vi "WM Period-Depth to Wave Length.vi"(1 "Water Depth":dbl=0.01 min=0.01 step=0.01 format="%.2f", 2 "Period":dbl=0.01 min=0.01 format="%.2f") -> (0 "WaveLength":dbl format="%.4f")   [LabVIEW 2012]
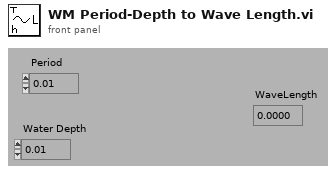
[diagram p1: front panel]
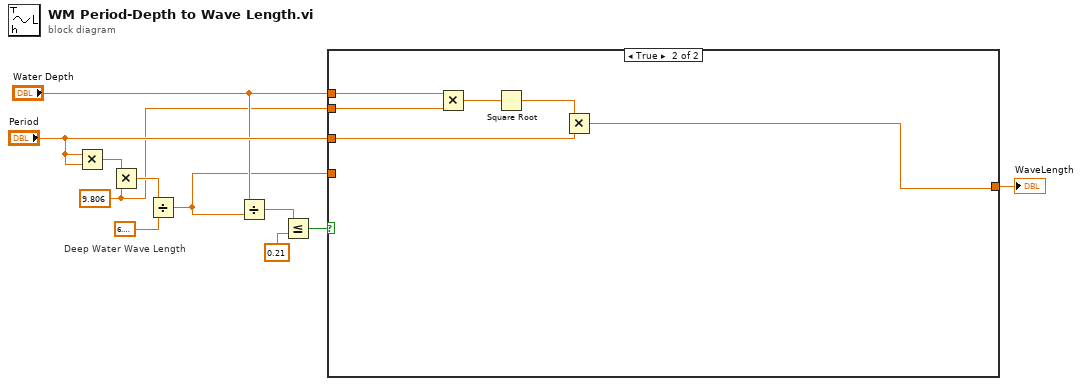
[diagram p0: block diagram]
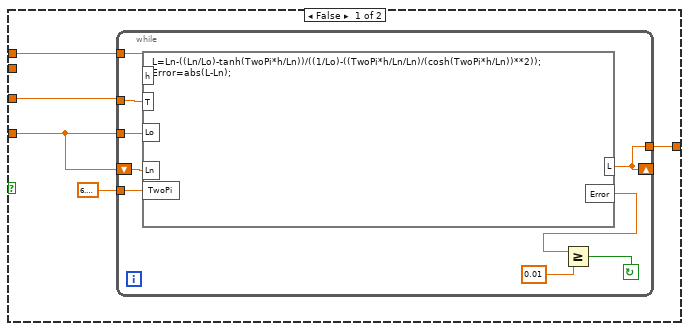
[diagram p2: hidden frame]
diagram:
  w1 = 9.806
  # "Deep Water Wave Length"
  n1 = Multiply(x="Period", y="Period") -> (x*y=w8:dbl)
  n2 = Multiply(x=w8, y=w1) -> (x*y=w10:dbl)
  n3 = Divide(x=w10, y=6.283185307179586) -> (x/y=w5:dbl)
  n4 = Divide(x="Water Depth", y=w5) -> (x/y=w4:dbl)
  n5 = Less Or Equal?(x=w4, y=0.21) -> (x <= y?=w2:bool)
  n6 = case shown="True" w2 {
    tunnel: "Water Depth" -> [w16 w30]
    tunnel: "Period" -> [w15 w31]
    tunnel: [w13 w27] -> w7
    tunnel: w5 -> [w12 _]
    tunnel: w1 -> [_ w26]
    frame False {
      n7 = while {
        tunnel: [w17] -> w13
        tunnel: 6.283185307179586 -> [w18]
        shift-left: w12 -> [w22]
        shift-right: [w17] -> _
        tunnel: w12 -> [w23]
        tunnel: w16 -> [w24]
        tunnel: w15 -> [w25]
        stop <- w19 continue-if-true
        n8 = formula code="L=Ln-((Ln/Lo)-tanh(TwoPi*h/Ln))/((1/Lo)-((TwoPi*h/Ln/Ln)/(cosh(TwoPi*h/Ln))**2));\nError=abs(L-Ln);"("T"=w25, "h"=w24, "Lo"=w23, "Ln"=w22, "TwoPi"=w18) -> ("L"=w17:dbl, "Error"=w21:dbl)
        n9 = Greater Or Equal?(x=w21, y=0.01) -> (x >= y?=w19:bool)
      }
    }
    frame True {
      n10 = Multiply(x=w30, y=w26) -> (x*y=w29:dbl)
      n11 = Square Root(x=w29) -> (sqrt(x)=w28:dbl)
      n12 = Multiply(x=w28, y=w31) -> (x*y=w27:dbl)
    }
  }
  "WaveLength" <- w7
